vi "read.vi"(0 "object in":refnum<class "MBinteractive.lvclass">, 1 "上次仪器状态":u16[](array[numeric]) caption="仪器状态", 2 "上次各参数测量间隔":u16[](array[numeric]) caption="各参数测量间隔", 5 "error in (no error)":errorcluster) -> (14 "object out":refnum<class "MBinteractive.lvclass">, 15 "仪器状态":u16[](array[numeric]), 17 "各参数测量间隔":u16[](array[numeric]), 19 "error out":errorcluster)   [LabVIEW 2016, in "MBinteractive.lvclass"]
uses:
  MBinteractive.lvclass
  <vilib>/NI/Modbus Library/API/Modbus API.lvclass
  <vilib>/ptbypt/NI_PtbyPt.lvlib
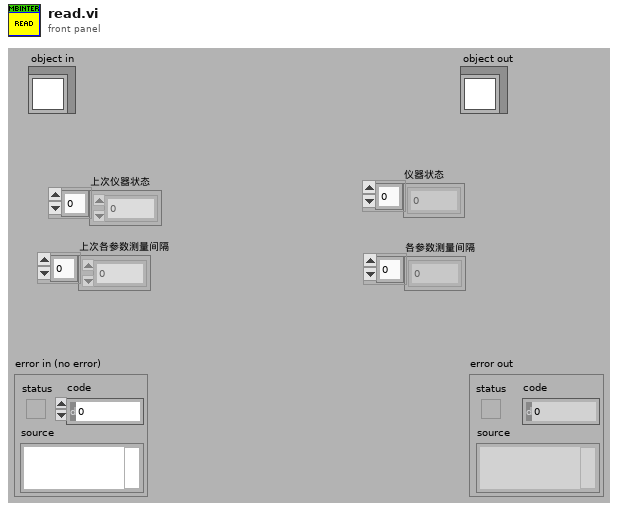
[diagram p1: front panel]
types:
  T1 = cluster{"系统状态":bool, "运行模式":bool, "测量周期":bool, "超标留样":bool, "反控数据":bool, "核查数据上传":bool, "实时小时数据上传":bool, "数据接收超时指示灯":bool, "数据发送起始时间":timestamp, "与工控软件通信":bool, "发送报文首页显示":string, "读取报文首页显示":string, "掉线指示灯":bool, "TCP掉线时间节点":string}
  T2 = cluster{"register values":u16[], "读取试剂余量的值":u16[], "读取各参数测量周期的值":u16[]}
  T3 = cluster{"[0]":bool, "[1]":bool, "[2]":bool, "[3]":bool, "[4]":bool}
  T4 = cluster{"[0]":bool, "[1]":bool, "[2]":bool, "[3]":bool, "[4]":bool, "[5]":bool}
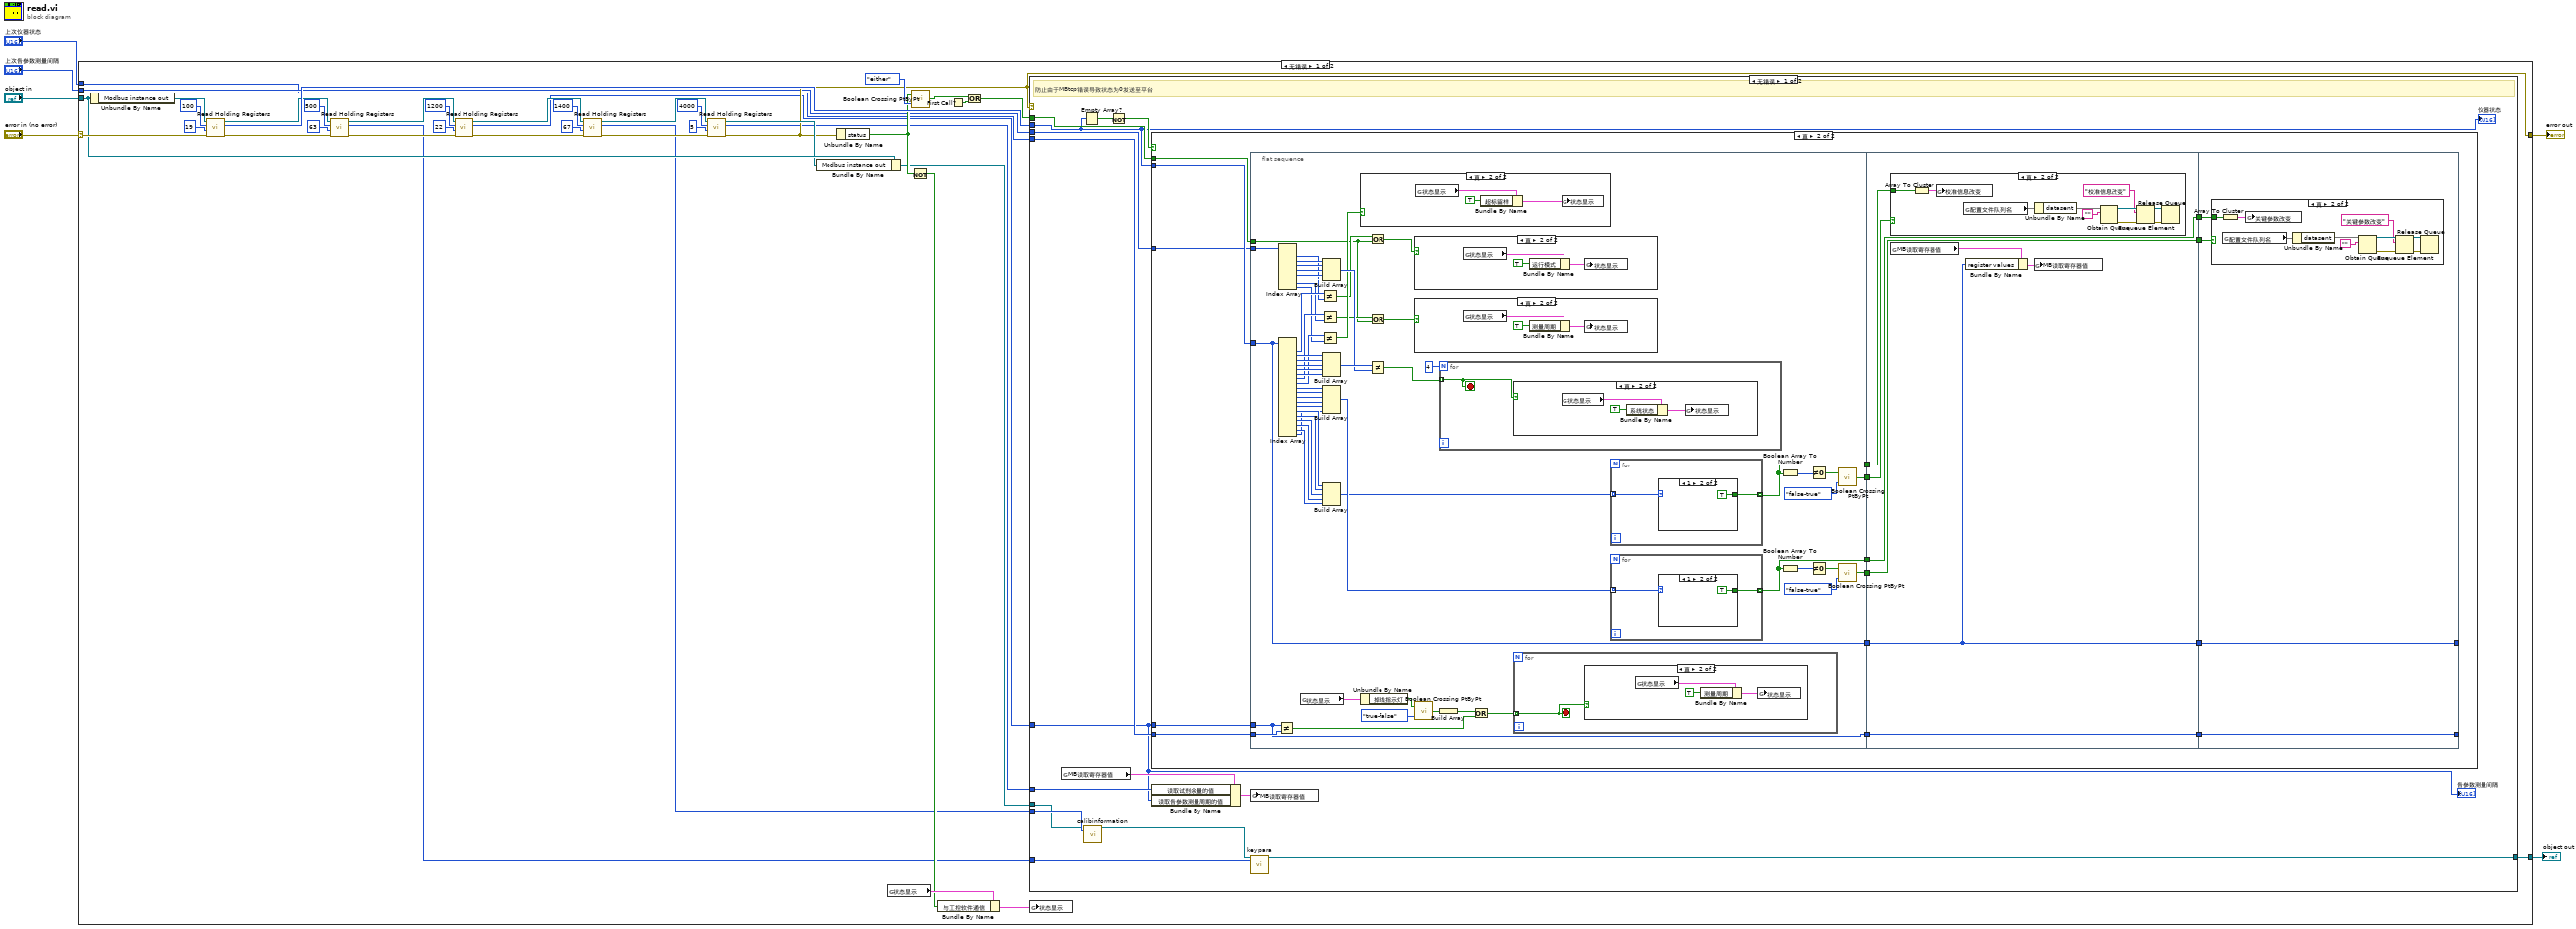
[diagram p0: block diagram]
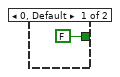
[diagram p3: hidden frame]
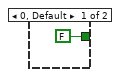
[diagram p4: hidden frame]
diagram:
  n1 = case shown="无错误" "error in (no error)" {
    selector: "error in (no error)" -> [w27 w196]
    tunnel: [w16 w196] -> w5
    tunnel: [w7 w195] -> w3
    tunnel: "object in" -> [w26 w195]
    tunnel: "上次仪器状态" -> [w10 _]
    tunnel: "上次各参数测量间隔" -> [w9 _]
    frame No Error {
      n2 = Unbundle By Name(w26) -> ("Modbus instance out"=w28:refnum<class "Modbus API.lvclass">)
      n3 = call-dynamic "Read Holding Registers.vi"("error in"=w27, "number of inputs"=u16 19 ("number of holding registers"), "starting address"=u16 100, "Modbus instance in"=w28) -> ("error out"=w17:errorcluster, "register values"=w44:u16[], "Modbus instance out"=w37:refnum<class "Modbus API.lvclass">)  [unwired: 5 in]
      n4 = call-dynamic "Read Holding Registers.vi"("error in"=w17, "number of inputs"=u16 63 ("number of holding registers"), "starting address"=u16 500, "Modbus instance in"=w37) -> ("error out"=w29:errorcluster, "register values"=w15:u16[], "Modbus instance out"=w36:refnum<class "Modbus API.lvclass">)  [unwired: 5 in]
      n5 = call-dynamic "Read Holding Registers.vi"("error in"=w29, "number of inputs"=u16 22 ("number of holding registers"), "starting address"=u16 1200, "Modbus instance in"=w36) -> ("error out"=w32:errorcluster, "register values"=w13:u16[], "Modbus instance out"=w33:refnum<class "Modbus API.lvclass">)  [unwired: 5 in]
      n6 = call-dynamic "Read Holding Registers.vi"("error in"=w32, "number of inputs"=u16 67 ("number of holding registers"), "starting address"=u16 1400, "Modbus instance in"=w33) -> ("error out"=w30:errorcluster, "register values"=w12:u16[], "Modbus instance out"=w31:refnum<class "Modbus API.lvclass">)  [unwired: 5 in]
      n7 = call-dynamic "Read Holding Registers.vi"("error in"=w30, "number of inputs"=u16 5 ("number of holding registers"), "starting address"=u16 4000, "Modbus instance in"=w31) -> ("error out"=w16:errorcluster, "register values"=w11:u16[], "Modbus instance out"=w25:refnum<class "Modbus API.lvclass">)  [unwired: 5 in]
      n8 = Bundle By Name(cluster=w26, "Modbus instance out"=w25) -> (w8:refnum<class "MBinteractive.lvclass">)
      n9 = Unbundle By Name(w16) -> ("status"=w14:bool)
      n10 = global read "全局1.vi" "状态显示"() -> (w23:T1)
      n11 = call <vilib>:"Boolean Crossing PtByPt.vi"("direction"=enum16{"either", "false-true", "true-false"}."either", "input"=w14) -> ("crossing"=w20:bool)  [unwired: 1 in]
      n12 = Not(x=w14) -> (.not. x?=w22:bool)
      n13 = Bundle By Name(cluster=w23, "与工控软件通信"=w22) -> (w24:T1)
      n14 = First Call?() -> (First Call?: T/F=w19:bool)
      n15 = Or(x=w20, y=w19) -> (x .or. y?=w18:bool)
      n16 = case shown="无错误" w16 {
        tunnel: w44 -> [w58 _]
        tunnel: w18 -> [w59 _]
        tunnel: w15 -> [w48 _]
        tunnel: w13 -> [w52 _]
        tunnel: w12 -> [w51 _]
        tunnel: w11 -> [w53 _]
        tunnel: w10 -> [w57 _]
        tunnel: w9 -> [w56 _]
        tunnel: w8 -> [w50 w194]
        tunnel: [w47 w194] -> w7
        frame No Error {
          # "防止由于MBtcp错误导致状态为0发送至平台"
          n17 = global read "全局1.vi" "MB读取寄存器值"() -> (w55:T2)
          n18 = Empty Array?(array=w58) -> (empty?=w61:bool)
          n19 = call-dynamic "calibinformation.vi"("object in"=w50, "校准点信息"=w51) -> ("object out"=w49:refnum<class "MBinteractive.lvclass">)  [unwired: 16 in, 1 out]
          n20 = Not(x=w61) -> (.not. x?=w60:bool)
          n21 = case shown="真" w60 {
            tunnel: w59 -> [_ w66]
            tunnel: w58 -> [_ w65]
            tunnel: w57 -> [_ w64]
            tunnel: w52 -> [_ w63]
            tunnel: w56 -> [_ w62]
            frame False {
            }
            frame True {
              n22 = flat-sequence {
                tunnel: w65 -> [w120]
                tunnel: [w120] -> w76
                tunnel: w64 -> [w116]
                tunnel: w66 -> [w111]
                tunnel: [w77] -> w75
                tunnel: w62 -> [w109]
                tunnel: [w98] -> w74
                tunnel: [w87] -> w73
                tunnel: [w86] -> w72
                tunnel: [w85] -> w71
                tunnel: w63 -> [w77]
                tunnel: w76 -> [w162]
                tunnel: w75 -> [w169]
                tunnel: w74 -> [w165]
                tunnel: w73 -> [w168]
                tunnel: w72 -> [w167]
                tunnel: w71 -> [w166]
                tunnel: [w162] -> w70
                tunnel: [w169] -> w69
                tunnel: [w166] -> w68
                tunnel: [w165] -> w67
                tunnel: [w182] -> _
                tunnel: [w183] -> _
                tunnel: w70 -> [w183]
                tunnel: w69 -> [w182]
                tunnel: w68 -> [w181]
                tunnel: w67 -> [w180]
                frame #0 {
                  n23 = Not Equal?(x=w77, y=w109) -> (x != y?=w108:bool[])
                  n24 = Index Array(array=w116) -> (element #1=w123:u16, element #2=w131:u16, element #3=w130:u16, element #4=w129:u16, element #5=w128:u16, element #6=w127:u16, element #7=w121:u16, element #8=w118:u16)  [unwired: 8 in]
                  n25 = Index Array(array=w120) -> (element #1=w124:u16, element #2=w136:u16, element #3=w135:u16, element #4=w134:u16, element #5=w133:u16, element #6=w132:u16, element #7=w122:u16, element #8=w119:u16, element #9=w106:u16, element #10=w105:u16, element #11=w104:u16, element #12=w103:u16, element #13=w102:u16, element #14=w96:u16, element #15=w95:u16, element #16=w94:u16, element #17=w93:u16, element #18=w92:u16, element #19=w80:u16)  [unwired: 19 in]
                  n26 = global read "全局1.vi" "状态显示"() -> (w79:T1)
                  n27 = Not Equal?(x=w124, y=w123) -> (x != y?=w114:bool)
                  n28 = Not Equal?(x=w122, y=w121) -> (x != y?=w112:bool)
                  n29 = Not Equal?(x=w119, y=w118) -> (x != y?=w117:bool)
                  n30 = Build Array(w131, w130, w129, w128, w127) -> (w125:u16[])
                  n31 = Build Array(w136, w135, w134, w133, w132) -> (w126:u16[])
                  n32 = Build Array(w106, w105, w104, w103, w102, w80) -> (w101:u16[])
                  n33 = Build Array(w96, w95, w94, w93, w92) -> (w88:u16[])
                  n34 = case shown="真" w117 {
                    frame False {
                    }
                    frame True {
                      n35 = global read "全局1.vi" "状态显示"() -> (w155:T1)
                      n36 = Bundle By Name(cluster=w155, "超标留样"=TRUE ("系统状态改变")) -> (w154:T1)
                      n37 = global write "全局1.vi" "状态显示"(w154) -> ()
                    }
                  }
                  n38 = Unbundle By Name(w79) -> ("掉线指示灯"=w78:bool)
                  n39 = Or(x=w114, y=w111) -> (x .or. y?=w113:bool)
                  n40 = Or(x=w112, y=w111) -> (x .or. y?=w110:bool)
                  n41 = Not Equal?(x=w126, y=w125) -> (x != y?=w115:bool[])
                  n42 = case shown="真" w113 {
                    frame False {
                    }
                    frame True {
                      n43 = global read "全局1.vi" "状态显示"() -> (w161:T1)
                      n44 = Bundle By Name(cluster=w161, "运行模式"=TRUE) -> (w160:T1)
                      n45 = global write "全局1.vi" "状态显示"(w160) -> ()
                    }
                  }
                  n46 = case shown="真" w110 {
                    frame False {
                    }
                    frame True {
                      n47 = global read "全局1.vi" "状态显示"() -> (w158:T1)
                      n48 = Bundle By Name(cluster=w158, "测量周期"=TRUE ("系统状态改变")) -> (w157:T1)
                      n49 = global write "全局1.vi" "状态显示"(w157) -> ()
                    }
                  }
                  n50 = call <vilib>:"Boolean Crossing PtByPt.vi"("direction"=enum16{"either", "false-true", "true-false"}."true-false", "input"=w78) -> ("crossing"=w82:bool)  [unwired: 1 in]
                  n51 = for {
                    N: 4 -> [_]
                    tunnel: w115 -> [w149] mode=indexing
                    stop <- w149 stop-if-true
                    n52 = case shown="真" w149 {
                      frame False {
                      }
                      frame True {
                        n53 = global read "全局1.vi" "状态显示"() -> (w152:T1)
                        n54 = Bundle By Name(cluster=w152, "系统状态"=TRUE ("系统状态改变")) -> (w151:T1)
                        n55 = global write "全局1.vi" "状态显示"(w151) -> ()
                      }
                    }
                  }
                  n56 = Build Array(w82) -> (w81:bool[])
                  n57 = Or(x=w81, y=w108) -> (x .or. y?=w84:bool[])
                  n58 = for {
                    tunnel: w84 -> [w145] mode=indexing
                    stop <- w145 stop-if-true
                    n59 = case shown="真" w145 {
                      frame False {
                      }
                      frame True {
                        n60 = global read "全局1.vi" "状态显示"() -> (w148:T1)
                        n61 = Bundle By Name(cluster=w148, "测量周期"=TRUE ("系统状态改变")) -> (w147:T1)
                        n62 = global write "全局1.vi" "状态显示"(w147) -> ()
                      }
                    }
                  }
                  n63 = for {
                    tunnel: w88 -> [w138] mode=indexing
                    tunnel: [w137] -> w86 mode=indexing
                    n64 = case shown="1" w138 {
                      tunnel: [FALSE TRUE] -> w137
                      frame 0, Default {
                      }
                      frame 1 {
                      }
                    }
                  }
                  n65 = for {
                    tunnel: w101 -> [w142] mode=indexing
                    tunnel: [w141] -> w85 mode=indexing
                    n66 = case shown="1" w142 {
                      tunnel: [FALSE TRUE] -> w141
                      frame 0, Default {
                      }
                      frame 1 {
                      }
                    }
                  }
                  n67 = Boolean Array To Number(Boolean array=w86) -> (number=w89:u32)
                  n68 = Boolean Array To Number(Boolean array=w85) -> (number=w100:u32)
                  n69 = Not Equal To 0?(x=w89) -> (x != 0?=w90:bool)
                  n70 = Not Equal To 0?(x=w100) -> (x != 0?=w99:bool)
                  n71 = call <vilib>:"Boolean Crossing PtByPt.vi"("direction"=enum16{"either", "false-true", "true-false"}."false-true", "input"=w90) -> ("crossing"=w87:bool)  [unwired: 1 in]
                  n72 = call <vilib>:"Boolean Crossing PtByPt.vi"("direction"=enum16{"either", "false-true", "true-false"}."false-true", "input"=w99) -> ("crossing"=w98:bool)  [unwired: 1 in]
                }
                frame #1 {
                  n73 = case shown="真" w168 {
                    tunnel: w167 -> [_ w172]
                    frame False {
                    }
                    frame True {
                      n74 = Array To Cluster(array=w172) -> (cluster=w171:T3)
                      n75 = global write "全局1.vi" "校准信息改变"(w171) -> ()
                      n76 = global read "断电保存全局.vi" "配置文件队列名"() -> (w170)
                      n77 = Unbundle By Name(w170) -> ("datasent"=w179)
                      n78 = Obtain Queue(name (unnamed)=w179, element data type="") -> (queue out=w177:refnum<queue>, error out=w175:errorcluster)  [unwired: 3 in, 1 out]
                      n79 = Enqueue Element(queue=w177, element="校准信息改变" ("元素"), error in (no error)=w175) -> (queue out=w174:refnum<queue>, error out=w173:errorcluster)  [unwired: 1 in, 1 out]
                      n80 = Release Queue(queue=w174, error in (no error)=w173) -> ()  [unwired: 1 in, 3 out]
                    }
                  }
                  n81 = global read "全局1.vi" "MB读取寄存器值"() -> (w164:T2)
                  n82 = Bundle By Name(cluster=w164, "register values"=w162) -> (w163:T2)
                  n83 = global write "全局1.vi" "MB读取寄存器值"(w163) -> ()
                }
                frame #2 {
                  n84 = case shown="真" w180 {
                    tunnel: w181 -> [_ w186]
                    frame False {
                    }
                    frame True {
                      n85 = Array To Cluster(array=w186) -> (cluster=w185:T4)
                      n86 = global read "断电保存全局.vi" "配置文件队列名"() -> (w184)
                      n87 = global write "全局1.vi" "关键参数改变"(w185) -> ()
                      n88 = Unbundle By Name(w184) -> ("datasent"=w193)
                      n89 = Obtain Queue(name (unnamed)=w193, element data type="") -> (queue out=w191:refnum<queue>, error out=w189:errorcluster)  [unwired: 3 in, 1 out]
                      n90 = Enqueue Element(queue=w191, element="关键参数改变" ("元素"), error in (no error)=w189) -> (queue out=w188:refnum<queue>, error out=w187:errorcluster)  [unwired: 1 in, 1 out]
                      n91 = Release Queue(queue=w188, error in (no error)=w187) -> ()  [unwired: 1 in, 3 out]
                    }
                  }
                }
              }
            }
          }
          n92 = Bundle By Name(cluster=w55, "读取试剂余量的值"=w53, "读取各参数测量周期的值"=w52) -> (w54:T2)
          n93 = global write "全局1.vi" "MB读取寄存器值"(w54) -> ()
          n94 = call-dynamic "keypara.vi"("object in"=w49, "关键参数"=w48) -> ("object out"=w47:refnum<class "MBinteractive.lvclass">)  [unwired: 16 in, 1 out]
          "仪器状态" <- w58
          "各参数测量间隔" <- w52
        }
        frame Error {
        }
      }
      n95 = global write "全局1.vi" "状态显示"(w24) -> ()
    }
    frame Error {
    }
  }
  "error out" <- w5
  "object out" <- w3
